vi "IMU.vi"() -> ()   [LabVIEW 2019]
uses:
  <vilib>/NI_Real-Time Target Support.lvlib
  <vilib>/Rock Robotics/SystemInterfaces/DIO/FPGA_DIOChannel.ctl
  <vilib>/Rock Robotics/SystemInterfaces/spilib/spi_bus.ctl
  <vilib>/Rock Robotics/WPI/SPI/WPI_SPIMode.ctl
  Downloads/ADIS16448-RoboRIO-Driver-master/ADIS16448-RoboRIO-Driver-master/LabVIEW/ADIS16448Lib/Typedef/ADIS16448 Hardware Configuration.ctl
  <vilib>/Utility/RT CPU Load.ctl
  Downloads/ADIS16448-RoboRIO-Driver-master/ADIS16448-RoboRIO-Driver-master/LabVIEW/ADIS16448Lib/Typedef/ADIS16448 Data.ctl
panel:
  out "IMU Detected?":bool
  out "Calibrated?":bool
  in  "Reset?":bool
  out "Integrated Gyro Angle":T1
  out "CPU loads":T2[](array[typedef]) {"ISR (%)" format="%#.2f"; "Idle (%)" format="%#.2f"; "Background (%)" format="%#.2f"; "Normal (%)" format="%#.2f"; "Above Normal (%)" format="%#.2f"; "High (%)" format="%#.2g"; "Timed Structures (%)" format="%#.2g"; "Time Critical (%)" format="%#.2g"; "Total (%)" format="%#.2g"}
  in  "Recalibrate":bool
  in  "Set Cal Time":bool
  in  "stop":bool
  in  "Hardware Config":T3={"SPI Clock Rate (Hz)"=1000000.0, "IMU SPI Mode (3)"=enum."Mode 3 (Clk Idle High,Sample on Trailing)", "IMU Reset Pin"=enum."DIO MXP 8", "IMU SPI Bus"=enum."SPI MXP", "IMU Data Ready Pin"=enum."DIO MXP 0", "Stall Config"={"Pow2BytesPerRead"=255, "StallTicks"=1000, "CsToSclkTicks"=100}, "IMU Status LED Pin"=enum."DIO MXP 9"}
  in  "Calibration Time (sec)":u32=4
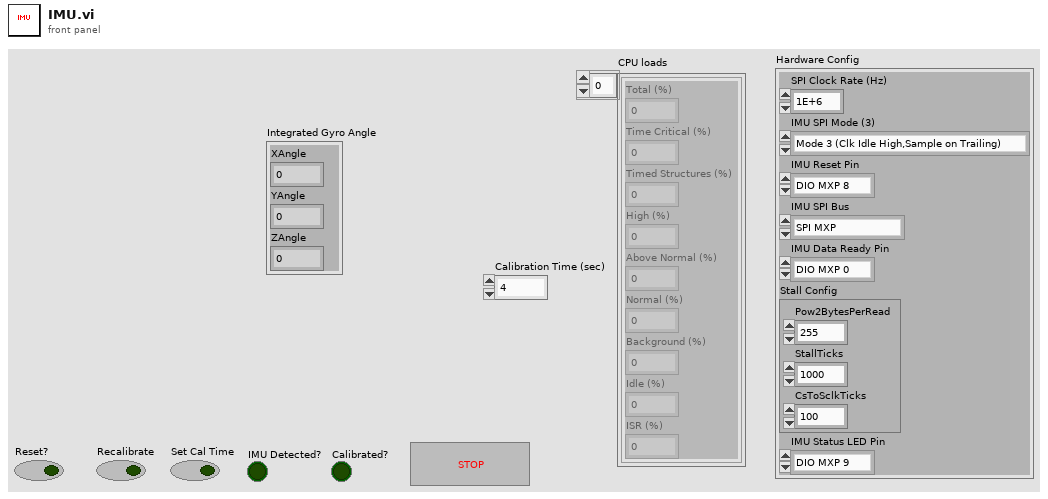
[diagram p1: front panel]
types:
  T1 = typedef "ADIS16448 Data.ctl" = cluster{"XAngle":dbl, "YAngle":dbl, "ZAngle":dbl}
  T2 = typedef "NI_Real-Time Target Support.lvlib/RT CPU Load.ctl" = cluster{"Total (%)":dbl, "Time Critical (%)":dbl, "Timed Structures (%)":dbl, "High (%)":dbl, "Above Normal (%)":dbl, "Normal (%)":dbl, "Background (%)":dbl, "Idle (%)":dbl, "ISR (%)":dbl}
  T3 = typedef "ADIS16448 Hardware Configuration.ctl" = cluster{"SPI Clock Rate (Hz)":dbl, "IMU SPI Mode (3)":T4, "IMU Reset Pin":T5, "IMU SPI Bus":T6, "IMU Data Ready Pin":T5, "Stall Config":cluster{"Pow2BytesPerRead":u8, "StallTicks":u16, "CsToSclkTicks":u8}, "IMU Status LED Pin":T5}
  T4 = typedef "WPI_SPIMode.ctl" = enum16{"Mode 0 (Clk Idle Low,Sample on Leading)", "Mode 1 (Clk Idle Low,Sample on Trailing)", "Mode 2 (Clk Idle High,Sample on Leading)", "Mode 3 (Clk Idle High,Sample on Trailing)"}
  T5 = typedef "FPGA_DIOChannel.ctl" = enum8{"DIO 0", "DIO 1", "DIO 2", "DIO 3", "DIO 4", "DIO 5", "DIO 6", "DIO 7", "DIO 8", "DIO 9", "DIO MXP 0", "DIO MXP 1", "DIO MXP 2", "DIO MXP 3", "DIO MXP 4", "DIO MXP 5", "DIO MXP 6", "DIO MXP 7", "DIO MXP 8", "DIO MXP 9", "DIO MXP 10", "DIO MXP 11", "DIO MXP 12", "DIO MXP 13", "DIO MXP 14", "DIO MXP 15", "SPI Port CS1", "SPI Port CS2", "SPI Port CS3", "SPI Port MISO", "SPI Port MOSI", "Invalid"}
  T6 = typedef "spi_bus.ctl" = enum16{"SPI On-Board, CS0", "SPI On-Board, CS1", "SPI On-Board, CS2", "SPI On-Board, CS3", "SPI MXP", "Invalid"}
  T7 = typedef "ADIS16448 Device Reference.ctl" = cluster{"DevStatus":errorcluster, "Hardware Config":T3, "Calibration Complete":refnum<notifier>, "Status FIFO":refnum<k33>, "Last Value Reference":refnum<data-value>, "Sychronous Process VI":T8, "Cmd FIFO":refnum<k33>, "Source":T9, "Data FIFO":refnum<k33>, "IMU Status LED Pin":T5, "Calibration Time":u32}
  T8 = typedef "ADIS16448 Process.ctl" = refnum<vi>
  T9 = typedef "FPGA_CounterEncoderSourceConvertionLVSourceType.ctl" = cluster{"DevStatus":errorcluster, "AnalogTriggerMode?":bool, "DigitalMode":cluster{"DIO Channel":T10}, "AnalogTriggerMode":cluster{"AnalogTriggerIndex":T11, "OutputType":T12}}
  T10 = typedef "FPGA_DIODigitalSourceChannel.ctl" = enum8{"DIO 0", "DIO 1", "DIO 2", "DIO 3", "DIO 4", "DIO 5", "DIO 6", "DIO 7", "DIO 8", "DIO 9", "DIO MXP 0", "DIO MXP 1", "DIO MXP 2", "DIO MXP 3", "DIO MXP 4", "DIO MXP 5", "DIO MXP 6", "DIO MXP 7", "DIO MXP 8", "DIO MXP 9", "DIO MXP 10", "DIO MXP 11", "DIO MXP 12", "DIO MXP 13", "DIO MXP 14", "DIO MXP 15", "SPI Port CS1", "SPI Port CS2", "SPI Port CS3", "SPI Port MISO", "SPI Port MOSI", "Disabled"}
  T11 = typedef "FPGA_AnalogTriggerIndex.ctl" = enum8{"Trig 0", "Trig 1", "Trig 2", "Trig 3", "Trig 4", "Trig 5", "Trig 6", "Trig 7", "Invalid"}
  T12 = typedef "FPGA_AnalogTriggerOutType.ctl" = enum16{"InWindow", "TriggerState", "Rising", "Falling"}
  T13 = typedef "ADIS16448 Status.ctl" = cluster{"Calibrated?":bool, "IMU Detected?":bool}
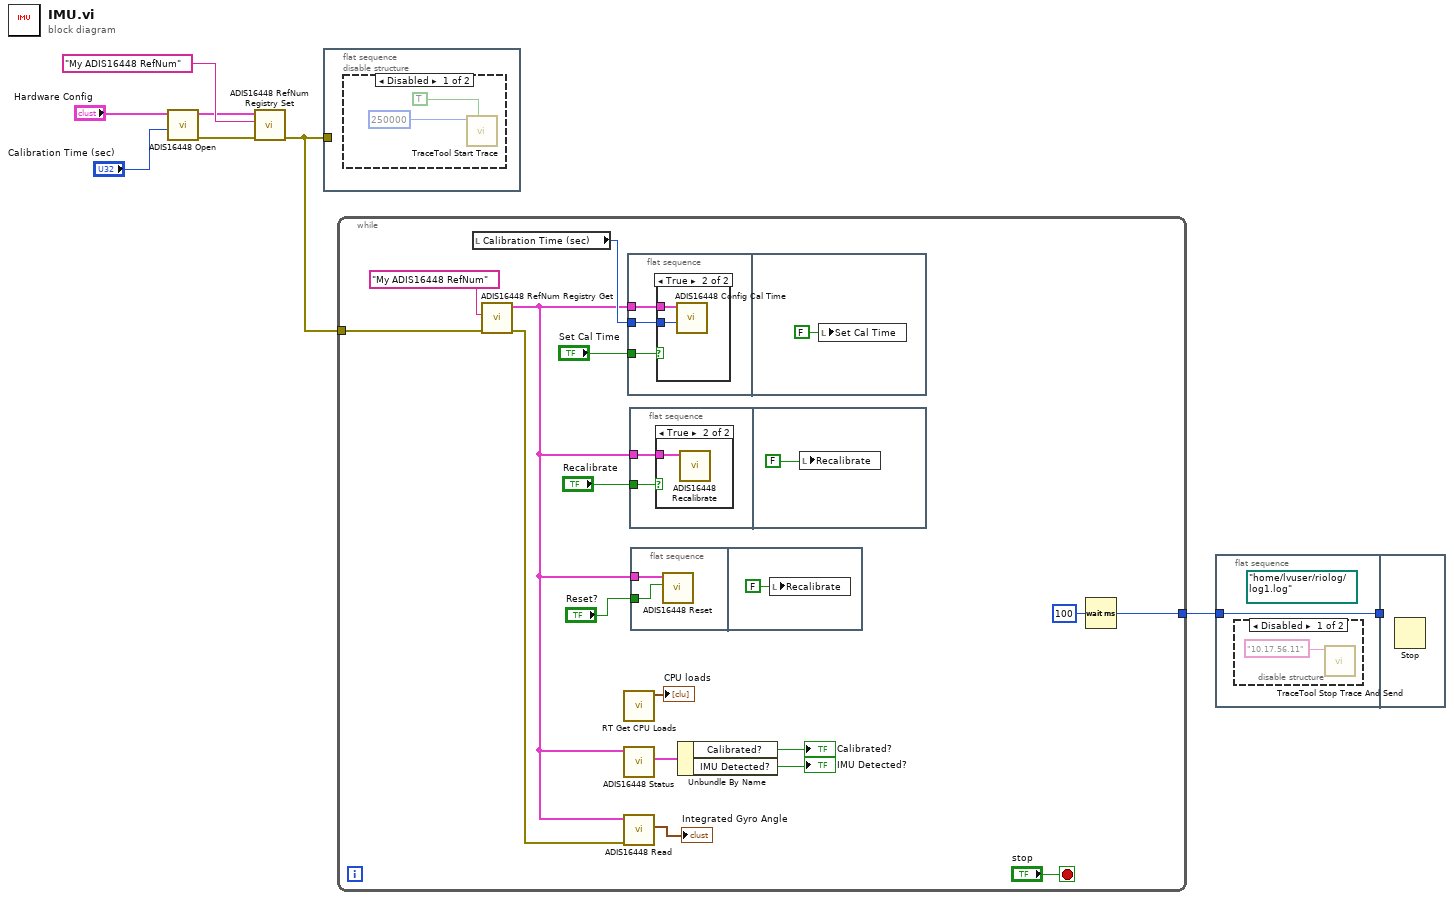
[diagram p0: block diagram]
diagram:
  n1 = call "ADIS16448 Open.vi"("Initial Calibration Time (sec)"="Calibration Time (sec)", "Hardware Config"="Hardware Config") -> ("error out"=w6:errorcluster, "ADIS16448DevRef"=w4:T7)  [unwired: 8 in]
  n2 = call "ADIS16448 RefNum Registry Set.vi"("error in (no error)"=w6, "refnum name"="My ADIS16448 RefNum", "ADIS16448DevRef"=w4) -> ("error out"=w3:errorcluster)  [unwired: 7 in, 1 out]
  n3 = flat-sequence {
    tunnel: w3 -> [_]
    frame #0 {
      n4 = disable-structure shown="Disabled" {
        frame Disabled {
          n5 = call <vilib>:"TraceTool Start Trace.vi"("Detailed Tracing? (F)"=TRUE, "Buffer Size (250000 bytes)"=250000) -> ()  [unwired: 8 in, 2 out]
        }
        frame Enabled {
        }
      }
    }
  }
  n6 = while {
    tunnel: w3 -> [w24]
    tunnel: [w11] -> w1
    stop <- "stop" stop-if-true
    n7 = local read "Calibration Time (sec)"() -> (w23:u32)
    n8 = call "ADIS16448 RefNum Registry Get.vi"("error in (no error)"=w24, "refnum name"="My ADIS16448 RefNum") -> ("error out"=w18:errorcluster, "ADIS16448DevRef Out"=w16:T7)  [unwired: 8 in]
    n9 = call <vilib>:"RT Get CPU Loads.vi"() -> ("CPU loads"=→"CPU loads":T2[])  [unwired: 10 in, 1 out]
    n10 = call "ADIS16448 Status.vi"("ADIS16448DevRef"=w16) -> ("ADIS16448 Status"=w15:T13)  [unwired: 8 in, 2 out]
    n11 = call "ADIS16448 Read.vi"("error in (no error)"=w18, "ADIS16448DevRef"=w16) -> ("ADIS16448 Value"=→"Integrated Gyro Angle":T1)  [unwired: 6 in, 3 out]
    n12 = flat-sequence {
      tunnel: w16 -> [w36]
      tunnel: w23 -> [w35]
      tunnel: "Set Cal Time" -> [w34]
      frame #0 {
        n13 = case shown="True" w34 {
          tunnel: w36 -> [_ w38]
          tunnel: w35 -> [_ w37]
          frame False {
          }
          frame True {
            n14 = call "ADIS16448 Config Cal Time.vi"("Data"=w37, "ADIS16448DevRef in"=w38) -> ()  [unwired: 8 in, 2 out]
          }
        }
      }
      frame #1 {
        n15 = local write "Set Cal Time"(FALSE ("Set Cal Time")) -> ()
      }
    }
    n16 = flat-sequence {
      tunnel: w16 -> [w31]
      tunnel: "Recalibrate" -> [w30]
      frame #0 {
        n17 = case shown="True" w30 {
          tunnel: w31 -> [_ w32]
          frame False {
          }
          frame True {
            n18 = call "ADIS16448 Recalibrate.vi"("ADIS16448DevRef in"=w32) -> ()  [unwired: 9 in, 2 out]
          }
        }
      }
      frame #1 {
        n19 = local write "Recalibrate"(FALSE ("Recalibrate")) -> ()
      }
    }
    n20 = flat-sequence {
      tunnel: "Reset?" -> [w28]
      tunnel: w16 -> [w27]
      frame #0 {
        n21 = call "ADIS16448 Reset.vi"("Reset?"=w28, "ADIS16448DevRef"=w27) -> ()  [unwired: 8 in, 2 out]
      }
      frame #1 {
        n22 = local write "Recalibrate"(FALSE ("Recalibrate")) -> ()
      }
    }
    n23 = Unbundle By Name(w15) -> ("Calibrated?"=→"Calibrated?":bool, "IMU Detected?"=→"IMU Detected?":bool)
    n24 = Wait (ms)(milliseconds to wait=u32 100) -> (millisecond timer value=w11:u32)
  }
  n25 = flat-sequence {
    tunnel: [w40] -> w2
    tunnel: w1 -> [w40]
    tunnel: w2 -> [_]
    frame #0 {
      (unwired) path "/home/lvuser/riolog/log1.log" ("Path to Trace Log")
      n26 = disable-structure shown="Disabled" {
        frame Disabled {
          n27 = call <vilib>:"TraceTool Stop Trace And Send.vi"("Trace Host Network Address"="10.17.56.11") -> ()  [unwired: 10 in, 1 out]
        }
        frame Enabled {
        }
      }
    }
    frame #1 {
      n28 = Stop() -> ()  [unwired: 1 in]
    }
  }
